vi "get_offset_pos.vi"(8 "error in (no error)":errorcluster caption="错误输入（无错误）", 10 "lab or motor":enum16{"lab", "motor"}(ring), 11 "OneMotion 输入":refnum<class "OneMotion.lvclass">) -> (0 "error out":errorcluster caption="错误输出", 1 "pos without offset":dbl, 2 "pos with offset":dbl, 3 "OneMotion 输出":refnum<class "OneMotion.lvclass">)   [LabVIEW 2016, in "MotionControl_UFO_3DOF.lvlib" / "OneMotion.lvclass"]
uses:
  <userlib>/MotionControl_UFO_3DOF/OneMotion/OneMotion.lvclass
  <userlib>/MotionControl_UFO_3DOF/OneMotion/OneMotion.lvclass/OneMotion.ctl
  <userlib>/MotionControl_UFO_3DOF/StepMotor/StepMotor.lvclass
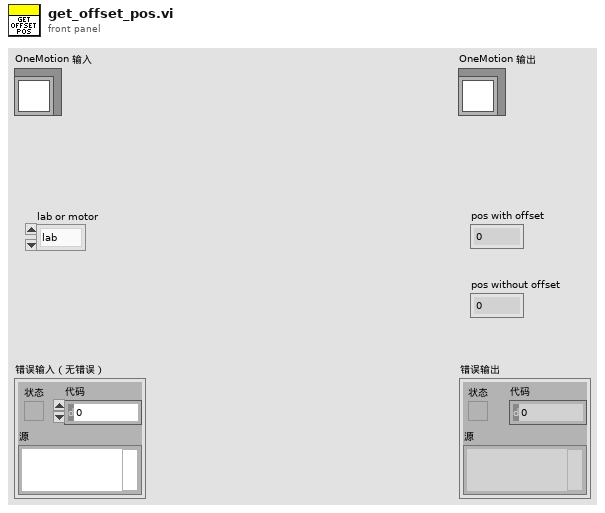
[diagram p1: front panel]
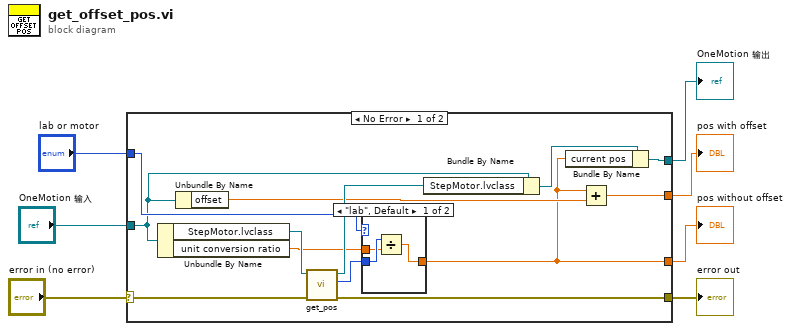
[diagram p0: block diagram]
diagram:
  n1 = case shown="No Error" "error in (no error)" {
    selector: "error in (no error)" -> [w18 w26]
    tunnel: [w8 w26] -> w6
    tunnel: [w13 w25] -> w4
    tunnel: "OneMotion 输入" -> [w15 w25]
    tunnel: "lab or motor" -> [w17 _]
    tunnel: [w12 _] -> w2
    tunnel: [w11 _] -> w1
    frame No Error {
      n2 = Unbundle By Name(w15) -> ("StepMotor.lvclass"=w20:refnum<class "StepMotor.lvclass">, "unit conversion ratio"=w10:dbl)
      n3 = Unbundle By Name(w15) -> ("offset"=w14:dbl)
      n4 = call-dynamic "get_pos.vi"("error in (no error)"=w18, "StepMotor 输入"=w20) -> ("error out"=w8:errorcluster, "pos"=w16:i32, "StepMotor 输出"=w19:refnum<class "StepMotor.lvclass">)  [unwired: 7 in]
      n5 = case shown="\"lab\", Default" w17 {
        tunnel: w16 -> [w23 w24]
        tunnel: [w21 w24] -> w11
        tunnel: w10 -> [w22 _]
        frame "lab", Default {
          n6 = Divide(x=w23, y=w22) -> (x/y=w21:dbl)
        }
        frame "motor" {
        }
      }
      n7 = Bundle By Name(cluster=w15, "StepMotor.lvclass"=w19) -> (w9:refnum<class "OneMotion.lvclass">)
      n8 = Bundle By Name(cluster=w9, "current pos"=w11) -> (w13:refnum<class "OneMotion.lvclass">)
      n9 = Add(x=w11, y=w14) -> (x+y=w12:dbl)
    }
    frame Error {
    }
  }
  "error out" <- w6
  "OneMotion 输出" <- w4
  "pos with offset" <- w2
  "pos without offset" <- w1
